vi "UDP Protocol FG.vi"(7 "Action":T1, 8 "error in (no error)":errorcluster, 10 "UDP Config":T2={"Local IP Address"="localhost", "Local Port"=8888, "Target IP Address"="localhost", "Target Port"=8888}, 11 "Device Item Ref in":T3 format="%.0x") -> (0 "error out":errorcluster, 2 "UDP Config":T2={"Local IP Address"="localhost", "Local Port"=8888, "Target IP Address"="localhost", "Target Port"=8888}, 3 "Item Ref out":T3 format="%.0x")   [LabVIEW 2020, in "Instrument Addon Shared.lvlib"]
uses:
  Instrument Addon Shared.lvlib
  <vilib>/NI VeriStand/Custom Device API/Custom Device Item Ref.ctl
  UDP Settings.ctl
  FG Control.ctl
  Constants.vi
  <vilib>/NI VeriStand/Custom Device API/Get Item Property (String).vi
  <vilib>/NI VeriStand/Custom Device API/Get Item Property (U32).vi
  <vilib>/NI VeriStand/Custom Device API/Set Item Property (String).vi
  <vilib>/NI VeriStand/Custom Device API/Set Item Property (U32).vi
  <vilib>/NI VeriStand/Custom Device API/Custom Device API.lvlib
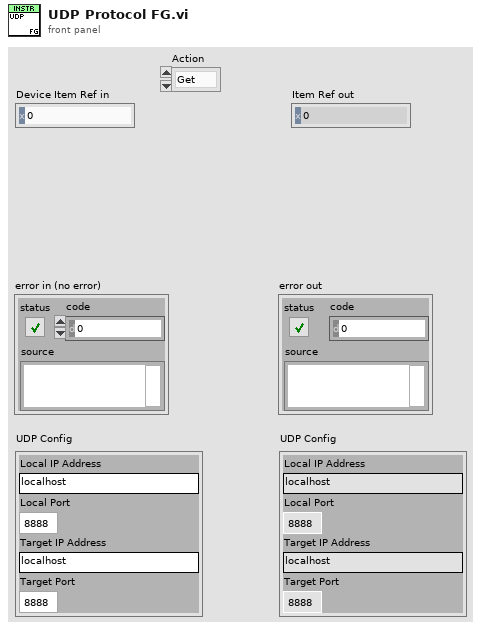
[diagram p1: front panel]
types:
  T1 = typedef "Instrument Addon Shared.lvlib/FG Control.ctl" = enum16{"Get", "Set"}
  T2 = typedef "Instrument Addon Shared.lvlib/UDP Settings.ctl" = cluster{"Local IP Address":string, "Local Port":u16, "Target IP Address":string, "Target Port":u16}
  T3 = typedef "Custom Device API.lvlib/Custom Device Item Ref.ctl" = u64
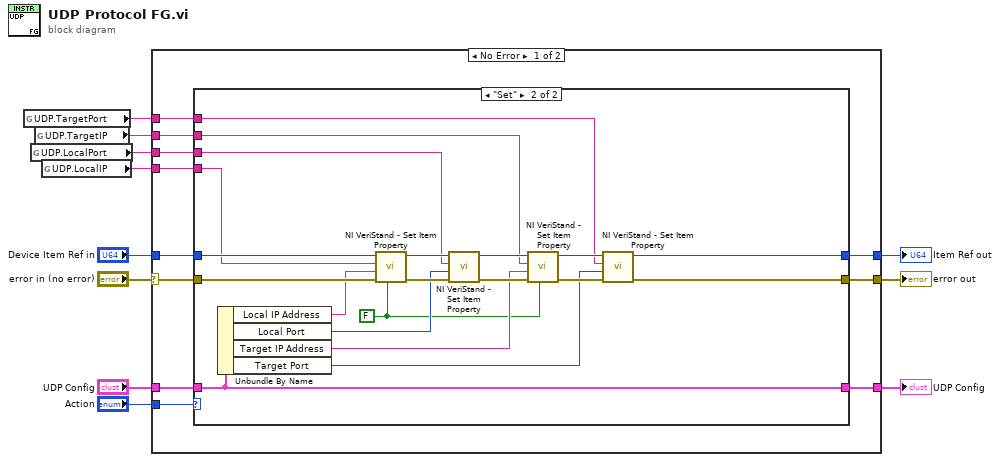
[diagram p0: block diagram]
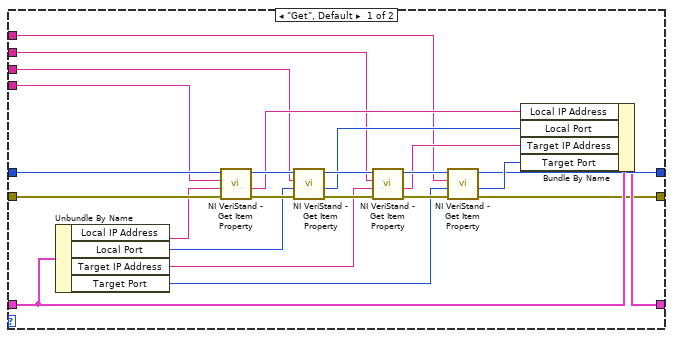
[diagram p2: hidden frame]
diagram:
  n1 = global read "Constants.vi" "UDP.TargetPort"() -> (w1:string)
  n2 = global read "Constants.vi" "UDP.LocalPort"() -> (w3:string)
  n3 = global read "Constants.vi" "UDP.TargetIP"() -> (w2:string)
  n4 = global read "Constants.vi" "UDP.LocalIP"() -> (w11:string)
  n5 = case shown="No Error" "error in (no error)" {
    selector: "error in (no error)" -> [w17 w69]
    tunnel: w11 -> [w22 _]
    tunnel: [w21 w67] -> w10
    tunnel: "Device Item Ref in" -> [w20 w67]
    tunnel: "UDP Config" -> [w19 w68]
    tunnel: [w18 w69] -> w7
    tunnel: [w16 w68] -> w5
    tunnel: "Action" -> [w15 _]
    tunnel: w3 -> [w14 _]
    tunnel: w2 -> [w13 _]
    tunnel: w1 -> [w12 _]
    frame No Error {
      n6 = case shown="\"Set\"" w15 {
        tunnel: w22 -> [w44 w56]
        tunnel: [w28 w58] -> w21
        tunnel: w20 -> [w45 w57]
        tunnel: w19 -> [w33 w52]
        tunnel: [w26 w59] -> w18
        tunnel: w17 -> [w46 w60]
        tunnel: [w27 w52] -> w16
        tunnel: w14 -> [w25 w55]
        tunnel: w13 -> [w24 w54]
        tunnel: w12 -> [w23 w53]
        frame "Get", Default {
          n7 = Unbundle By Name(w33) -> ("Local IP Address"=w37:string, "Local Port"=w36:u16, "Target IP Address"=w35:string, "Target Port"=w34:u16)
          n8 = call-poly <vilib>:"NI VeriStand - Get Item Property.vi"("error in (no error)"=w46, "Default Value"=w37, "Property Name"=w44, "Item Ref in"=w45) -> ("error out"=w43:errorcluster, "Value"=w32:string, "Item Ref out"=w42:T3)  [unwired: 4 in, 1 out]
          n9 = call-poly <vilib>:"NI VeriStand - Get Item Property.vi"("error in (no error)"=w43, "Default Value"=w36, "Property Name"=w25, "Item Ref in"=w42) -> ("error out"=w39:errorcluster, "Value"=w31:u32, "Item Ref out"=w41:T3)  [unwired: 4 in, 1 out]
          n10 = call-poly <vilib>:"NI VeriStand - Get Item Property.vi"("error in (no error)"=w39, "Default Value"=w35, "Property Name"=w24, "Item Ref in"=w41) -> ("error out"=w38:errorcluster, "Value"=w30:string, "Item Ref out"=w40:T3)  [unwired: 4 in, 1 out]
          n11 = call-poly <vilib>:"NI VeriStand - Get Item Property.vi"("error in (no error)"=w38, "Default Value"=w34, "Property Name"=w23, "Item Ref in"=w40) -> ("error out"=w26:errorcluster, "Value"=w29:u32, "Item Ref out"=w28:T3)  [unwired: 4 in, 1 out]
          n12 = Bundle By Name(cluster=w33, "Local IP Address"=w32, "Local Port"=w31, "Target IP Address"=w30, "Target Port"=w29) -> (w27:T2)
        }
        frame "Set" {
          w47 = FALSE ("Binary String (T)")
          n13 = Unbundle By Name(w52) -> ("Local IP Address"=w51:string, "Local Port"=w50:u16, "Target IP Address"=w49:string, "Target Port"=w48:u16)
          n14 = call-poly <vilib>:"NI VeriStand - Set Item Property.vi"("Binary String (T)"=w47, "error in (no error)"=w60, "Value"=w51, "Property Name"=w56, "Item Ref in"=w57) -> ("error out"=w66:errorcluster, "Item Ref out"=w65:T3)  [unwired: 4 in, 1 out]
          n15 = call-poly <vilib>:"NI VeriStand - Set Item Property.vi"("error in (no error)"=w66, "Value"=w50, "Property Name"=w55, "Item Ref in"=w65) -> ("error out"=w62:errorcluster, "Item Ref out"=w64:T3)  [unwired: 5 in, 1 out]
          n16 = call-poly <vilib>:"NI VeriStand - Set Item Property.vi"("Binary String (T)"=w47, "error in (no error)"=w62, "Value"=w49, "Property Name"=w54, "Item Ref in"=w64) -> ("error out"=w61:errorcluster, "Item Ref out"=w63:T3)  [unwired: 4 in, 1 out]
          n17 = call-poly <vilib>:"NI VeriStand - Set Item Property.vi"("error in (no error)"=w61, "Value"=w48, "Property Name"=w53, "Item Ref in"=w63) -> ("error out"=w59:errorcluster, "Item Ref out"=w58:T3)  [unwired: 5 in, 1 out]
        }
      }
    }
    frame Error {
    }
  }
  "Item Ref out" <- w10
  "error out" <- w7
  "UDP Config" <- w5
